vi "Create Mapper VIs for Enum.vi"(8 "error in (no error)":errorcluster, 10 "RPC Message Name":string, 11 "Library item in":refnum<vi>) -> (0 "error out":errorcluster, 3 "Library item out":refnum<vi>)   [LabVIEW 2019, in "gRPC Template Creation Utility.lvlib"]
uses:
  gRPC Template Creation Utility.lvlib
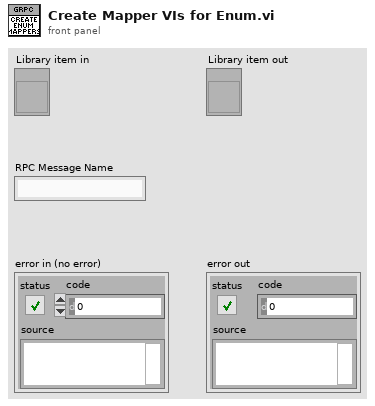
[diagram p1: front panel]
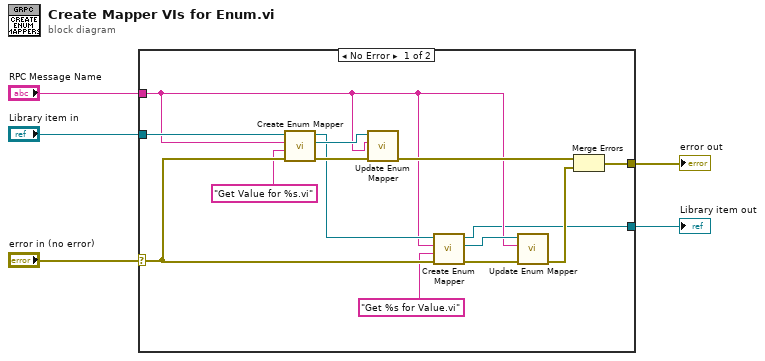
[diagram p0: block diagram]
diagram:
  n1 = case shown="No Error" "error in (no error)" {
    selector: "error in (no error)" -> [w16 w21]
    tunnel: "RPC Message Name" -> [w7 _]
    tunnel: [w13 w21] -> w4
    tunnel: "Library item in" -> [w17 w20]
    tunnel: [w6 w20] -> w1
    frame No Error {
      n2 = call "Create Enum Mapper.vi"("error in"=w16, "format string"="Get Value for %s.vi", "RPC Message Name"=w7, "Library item in"=w17) -> ("error out"=w19:errorcluster, "VI out"=w10:refnum<vi>, "Library item out"=w9:refnum<vi>)  [unwired: 5 in]
      n3 = call "Update Enum Mapper.vi"("error in"=w19, "RPC Message Name"=w7, "VI in"=w10) -> ("error out"=w15:errorcluster)  [unwired: 8 in]
      n4 = call "Create Enum Mapper.vi"("error in"=w16, "format string"="Get %s for Value.vi", "RPC Message Name"=w7, "Library item in"=w9) -> ("error out"=w18:errorcluster, "VI out"=w8:refnum<vi>, "Library item out"=w6:refnum<vi>)  [unwired: 5 in]
      n5 = call "Update Enum Mapper.vi"("error in"=w18, "RPC Message Name"=w7, "VI in"=w8) -> ("error out"=w14:errorcluster)  [unwired: 8 in]
      n6 = Merge Errors(w15, w14) -> (w13:errorcluster)
    }
    frame Error {
    }
  }
  "error out" <- w4
  "Library item out" <- w1
